vi "WaitForNewLocalization.vi"() -> (0 "Localization Status":T1)   [LabVIEW 2015]
doc: "Blocks until a new localization reading comes in, and returns it."
uses:
  LocalizationStatus.ctl
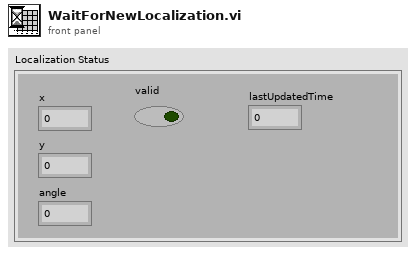
[diagram p1: front panel]
types:
  T1 = typedef "LocalizationStatus.ctl" = cluster{"x":dbl, "y":dbl, "angle":dbl, "valid":bool, "lastUpdatedTime":dbl}
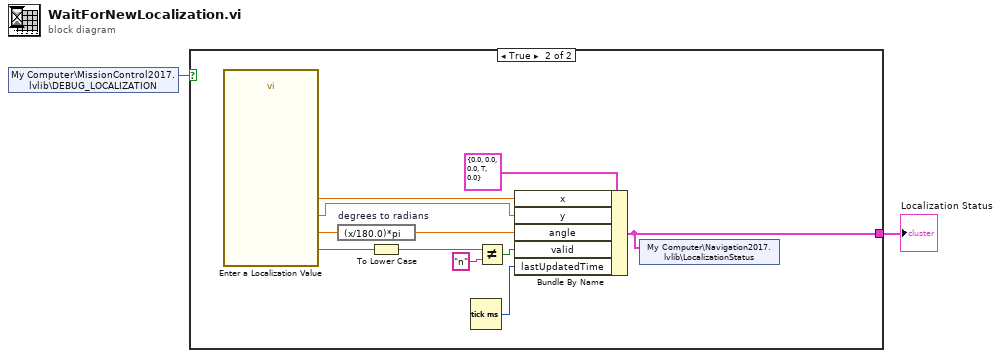
[diagram p0: block diagram]
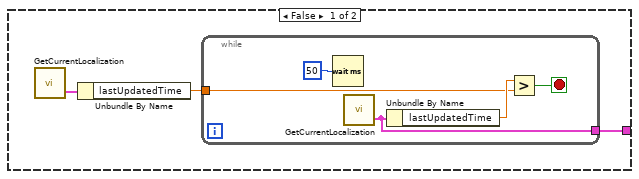
[diagram p2: hidden frame]
diagram:
  n1 = shared-variable "My Computer\\MissionControl2017.lvlib\\DEBUG_LOCALIZATION"() -> (w1:bool)  [unwired: 1 in, 1 out]
  n2 = case shown="True" w1 {
    tunnel: [w4 w20] -> w2
    frame False {
      n3 = call "GetCurrentLocalization.vi"() -> ("Current Localization Status"=w3:T1)  [unwired: 1 out]
      n4 = Unbundle By Name(w3) -> ("lastUpdatedTime"=w5:dbl)
      n5 = while {
        tunnel: w5 -> [w9]
        tunnel: [w6] -> w4
        stop <- w8 stop-if-true
        n6 = Wait (ms)(milliseconds to wait=u32 50) -> ()  [unwired: 1 out]
        n7 = call "GetCurrentLocalization.vi"() -> ("Current Localization Status"=w6:T1)  [unwired: 1 out]
        n8 = Unbundle By Name(w6) -> ("lastUpdatedTime"=w10:dbl)
        n9 = Greater?(x=w10, y=w9) -> (0:w8:bool)
      }
    }
    frame True {
      n10 = call "Enter a Localization Value"() -> ("valid? (Y/n)"=w13:string, "angle (deg)"=w16:dbl, "y (m)"=w18:dbl, "x (m)"=w19:dbl)  [unwired: 14 in, 2 out]
      n11 = expression code="(x/180.0)*pi" "degrees to radians"(w16) -> (w17:dbl)
      n12 = To Lower Case(string=w13) -> (all lower case string=w15:string)
      n13 = Tick Count (ms)() -> (millisecond timer value=w11:u32)
      n14 = Not Equal?(x=w15, y="n") -> (x != y?=w12:bool)
      n15 = Bundle By Name(cluster=T1 {"x"=0.0, "y"=0.0, "angle"=0.0, "valid"=TRUE, "lastUpdatedTime"=0.0} ("Localization Status"), "x"=w19, "y"=w18, "angle"=w17, "valid"=w12, "lastUpdatedTime"=w11) -> (w20:T1)
      n16 = shared-variable "My Computer\\Navigation2017.lvlib\\LocalizationStatus"(w20) -> ()  [unwired: 1 in, 1 out]
    }
  }
  "Localization Status" <- w2
